vi "Measurement.IVCurve.GetStaticDependencies.vi"(8 "error in (no error)":errorcluster, 11 "Measurement.IVCurve in":refnum<class "Measurement.IVCurve.lvclass">) -> (0 "error out":errorcluster, 2 "Dependencies":T1, 3 "Measurement.IVCurve out":refnum<class "Measurement.IVCurve.lvclass">)   [LabVIEW 2017, in "Measurement.IVCurve.lvclass"]
uses:
  Measurement.IVCurve.lvclass
  D:/Program Files (x86)/National Instruments/LabVIEW 2017/vi.lib/JKI/JKI SMO/SMO/SMO.lvclass
  Typedefs/Dependencies--Cluster.ctl
  SMU/SMU.lvclass
  <vilib>/JKI/JKI SMO/SMO/SMO.lvclass
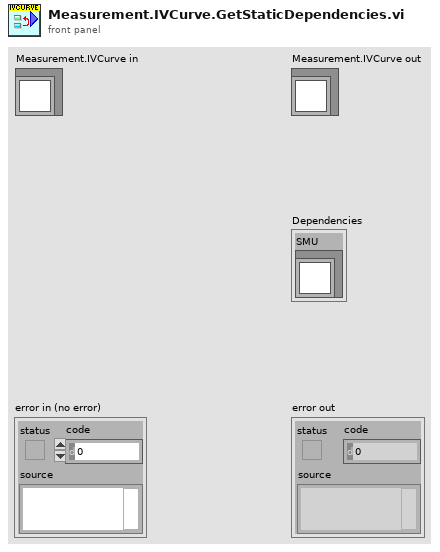
[diagram p1: front panel]
types:
  T1 = typedef "Measurement.IVCurve.lvclass/Dependencies--Cluster.ctl" = cluster{"SMU":refnum<class "SMU.lvclass">}
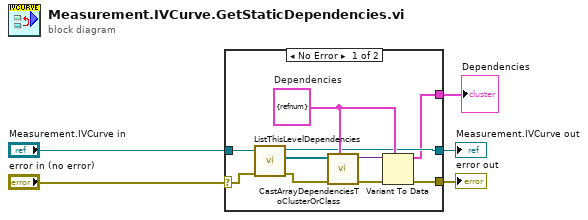
[diagram p0: block diagram]
diagram:
  n1 = case shown="No Error" "error in (no error)" {
    selector: "error in (no error)" -> [w14 w17]
    tunnel: [w8 w17] -> w4
    tunnel: [w7 w16] -> w2
    tunnel: "Measurement.IVCurve in" -> [w15 w16]
    tunnel: [w6 _] -> w1
    frame No Error {
      w9 = T1 {"SMU"=refnum}  # Dependencies
      n2 = call <vilib>:"ListThisLevelDependencies.vi"("error in (no error)"=w14, "SMO in"=w15) -> ("error out"=w12:errorcluster, "[My Dependencies]"=w13:refnum<class "SMO.lvclass">[], "SMO out"=w7:refnum<class "Measurement.IVCurve.lvclass">)  [unwired: 7 in]
      n3 = call <vilib>:"CastArrayDependenciesToClusterOrClass.vi"("Dependency Type (Class|Cluster)"=w9, "error in (no error)"=w12, "[Dependencies]"=w13) -> ("error out"=w11:errorcluster, "Dependencies output"=w10:variant)  [unwired: 7 in]
      n4 = Variant To Data(error in=w11, type=w9, Variant=w10) -> (data=w6:T1, error out=w8:errorcluster)
    }
    frame Error {
    }
  }
  "error out" <- w4
  "Measurement.IVCurve out" <- w2
  "Dependencies" <- w1
